vi "updateSuccesfulTimer.vi"(8 "error in (no error)":errorcluster, 11 "deviceHeartbeat in":refnum<class "deviceHeartbeat.lvclass">) -> (0 "error out":errorcluster, 3 "deviceHeartbeat out":refnum<class "deviceHeartbeat.lvclass">)   [LabVIEW 2016, in "deviceHeartbeat.lvclass"]
uses:
  deviceHeartbeat.lvclass
  deviceHeartbeat.lvclass/deviceHeartbeat.ctl
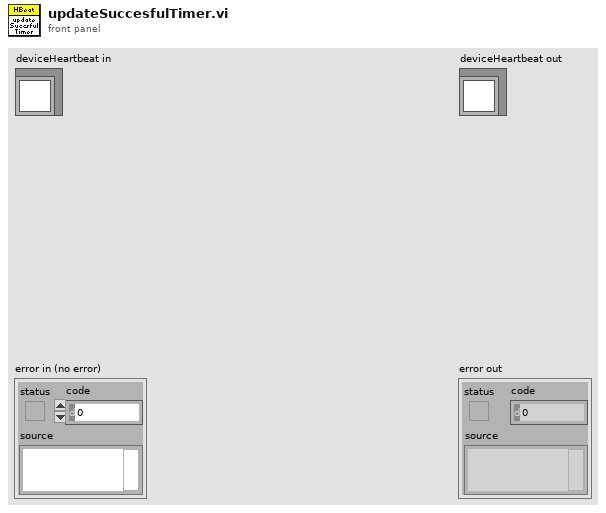
[diagram p1: front panel]
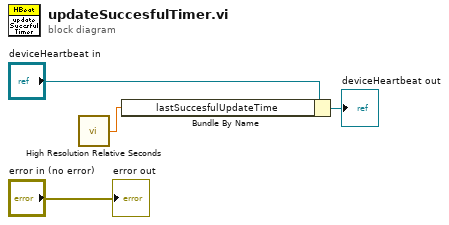
[diagram p0: block diagram]
diagram:
  n1 = call <vilib>:"High Resolution Relative Seconds.vi"() -> ("relative seconds"=w3:dbl)
  n2 = Bundle By Name(cluster="deviceHeartbeat in", "lastSuccesfulUpdateTime"=w3) -> (→"deviceHeartbeat out":refnum<class "deviceHeartbeat.lvclass">)
  "error out" <- "error in (no error)"
